vi "F to C (SUB VI).vi"(1 "Boolean":bool, 2 "Farenheit":dbl) -> (0 "Celcius":dbl)   [LabVIEW 2012]
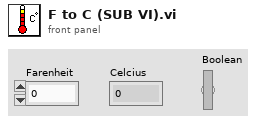
[diagram p1: front panel]
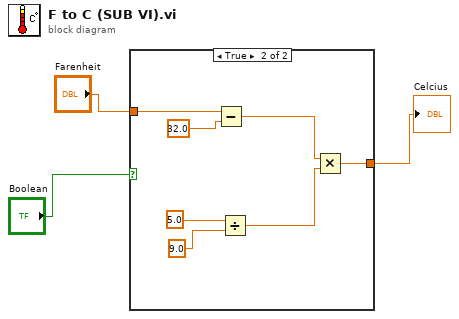
[diagram p0: block diagram]
diagram:
  n1 = case shown="True" "Boolean" {
    tunnel: [w4 w11] -> w3
    tunnel: "Farenheit" -> [w4 w5]
    frame False {
    }
    frame True {
      n2 = Subtract(x=w5, y=32.0 ("Thermometer")) -> (x-y=w9:dbl)
      n3 = Divide(x=5.0 ("Thermometer"), y=9.0 ("Thermometer")) -> (x/y=w10:dbl)
      n4 = Multiply(x=w9, y=w10) -> (x*y=w11:dbl)
    }
  }
  "Celcius" <- w3
